vi "get_buoy_coords.vi"(8 "error in (no error)":errorcluster, 11 "round_buoy in":refnum<class "round_buoy.lvclass">) -> (0 "error out":errorcluster, 2 "Buoy Coords":cluster{"X":dbl, "Y":dbl}, 3 "round_buoy out":refnum<class "round_buoy.lvclass">)   [LabVIEW 2011, in "round_buoy.lvclass"]
uses:
  round_buoy.lvclass
  round_buoy.lvclass/round_buoy.ctl
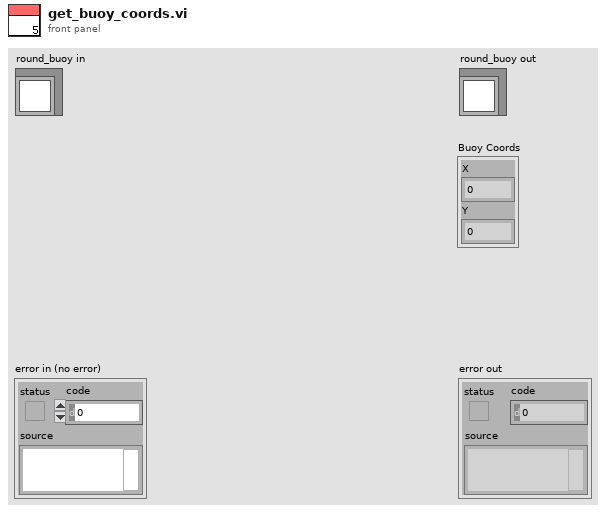
[diagram p1: front panel]
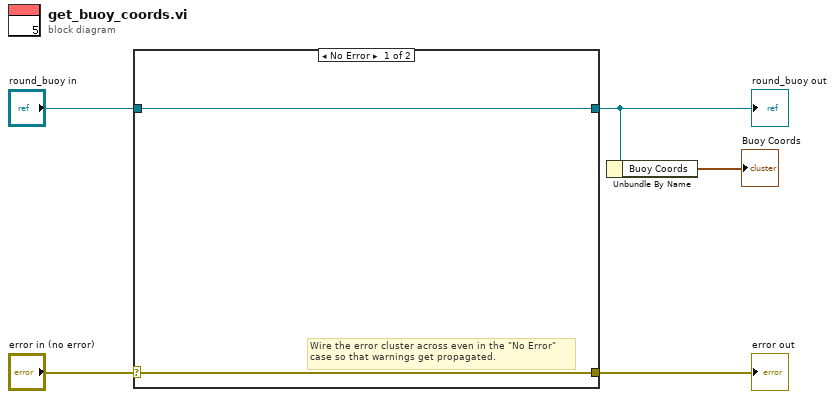
[diagram p0: block diagram]
diagram:
  n1 = case shown="No Error" "error in (no error)" {
    selector: "error in (no error)" -> [w6 w9]
    tunnel: [w6 w9] -> w4
    tunnel: [w7 w8] -> w2
    tunnel: "round_buoy in" -> [w7 w8]
    frame No Error {
      # "Wire the error cluster across even in the \"No Error\"\ncase so that warnings get propagated."
    }
    frame Error {
    }
  }
  "error out" <- w4
  "round_buoy out" <- w2
  n2 = Unbundle By Name(w2) -> ("Buoy Coords"=→"Buoy Coords":cluster{"X":dbl, "Y":dbl})
